vi "Transform.vi"(8 "error in (no error)":errorcluster caption="entrée d'erreur (pas d'erreur)", 9 "y":string[][](array[string]), 10 "X":string[][](array[string]), 11 "KNNImputer.lvclass":refnum<class "KNNImputer.lvclass">) -> (0 "error out":errorcluster caption="sortie d'erreur", 2 "Data":T1, 3 "KNNImputer.lvclass":refnum<class "KNNImputer.lvclass">)   [LabVIEW 2020, in "KNNImputer.lvclass"]
doc: "Impute all missing values in X.\n\nReturns : \n\n- X : array-like of shape (n_samples, n_output_features)\nThe imputed dataset. n_output_features is the number of features that is not always missing during fit."
uses:
  KNNImputer.lvclass
  KNNImputer.lvclass/KNNImputer.ctl
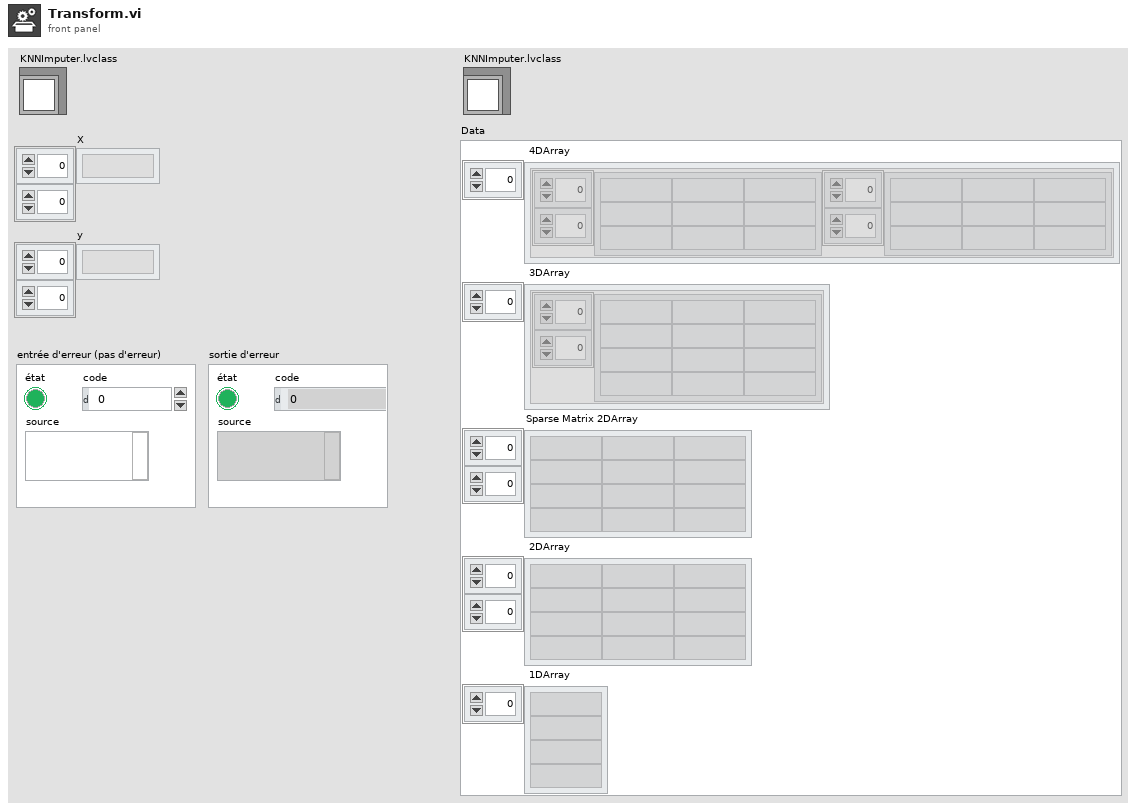
[diagram p1: front panel]
types:
  T1 = cluster{" 4DArray":cluster{"1":string[][], "2":string[][]}[], " 3DArray":cluster{"Tableau":string[][]}[], "Sparse Matrix 2DArray":string[][], " 2DArray":string[][], " 1DArray":string[]}
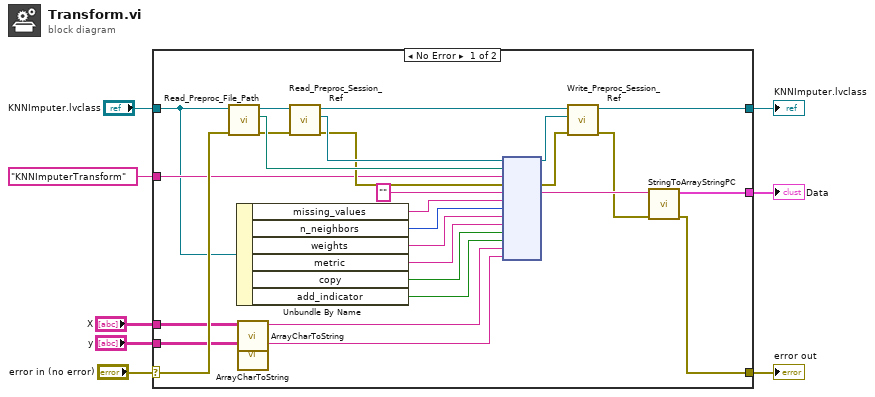
[diagram p0: block diagram]
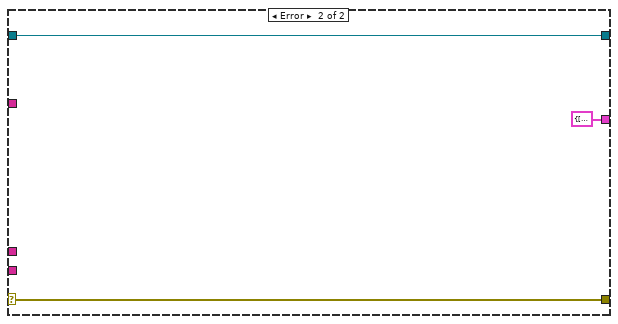
[diagram p2: hidden frame]
diagram:
  n1 = case shown="No Error" "error in (no error)" {
    selector: "error in (no error)" -> [w26 w38]
    tunnel: [w13 w38] -> w7
    tunnel: [w17 w37] -> w5
    tunnel: "KNNImputer.lvclass" -> [w24 w37]
    tunnel: "KNNImputerTransform" ("Fonction") -> [w25 _]
    tunnel: [w15 T1 {" 4DArray"=[], " 3DArray"=[], "Sparse Matrix 2DArray"=[], " 2DArray"=[], " 1DArray"=[]} ("Data")] -> w1
    tunnel: "X" -> [w12 _]
    tunnel: "y" -> [w10 _]
    frame No Error {
      n2 = call-dynamic "Read_Preproc_File_Path.vi"("error in (no error)"=w26, "Python in"=w24) -> ("error out"=w30:errorcluster, "File_Path"=w33:path, "Python out"=w35:refnum<class "KNNImputer.lvclass">)  [unwired: 7 in]
      n3 = Unbundle By Name(w24) -> ("missing_values"=w23:string, "n_neighbors"=w22:i32, "weights"=w21:string, "metric"=w20:string, "copy"=w19:bool, "add_indicator"=w18:bool)
      n4 = call "ArrayCharToString.vi"("TAB"=w12) -> ("Instruction"=w11:string)  [unwired: 10 in]
      n5 = call "ArrayCharToString.vi"("TAB"=w10) -> ("Instruction"=w9:string)  [unwired: 10 in]
      n6 = call-dynamic "Read_Preproc_Session_Ref.vi"("error in (no error)"=w30, "Python in"=w35) -> ("error out"=w31:errorcluster, "Session_ref"=w32:refnum<k35>, "Python out"=w34:refnum<class "KNNImputer.lvclass">)  [unwired: 7 in]
      n7 = node(w32, w33, w25, w31, "", w23, w22, w21, w20, w19, w18, w11, w9) -> (w27:refnum<k35>, w29:errorcluster, w16:string)  [unwired: 8 in, 2 out]
      n8 = call-dynamic "Write_Preproc_Session_Ref.vi"("error in (no error)"=w29, "Session_ref"=w27, "Python in"=w34) -> ("error out"=w14:errorcluster, "Python out"=w17:refnum<class "KNNImputer.lvclass">)  [unwired: 7 in]
      n9 = call "StringToArrayStringPC.vi"("sortie d'erreur"=w14, "Return value"=w16) -> ("sortie d'erreur"=w13:errorcluster, "Data"=w15:T1)  [unwired: 8 in]
    }
    frame Error {
    }
  }
  "error out" <- w7
  "KNNImputer.lvclass" <- w5
  "Data" <- w1
